vi "Configure Continuity.vi"(0 "VISA resource name":refnum<visa-resource-name>, 5 "Threshold (10)":dbl=10.0, 11 "error in (no error)":errorcluster) -> (4 "VISA resource name out":refnum<visa-resource-name>, 15 "error out":errorcluster)   [LabVIEW 2020, in "Keithley 27XX.lvlib"]
doc: "This VI configures the hreshold for continuity measurements.\n\nNote: \n(1) Configure Measurement.vi must be called <B>before</B> setting the threshold.\n\n(2) This VI will only work in Continuity Measurement mode.\n\n(3) This VI configures a global setting. Therefore, this VI does not require a scan list."
uses:
  Keithley 27XX.lvlib
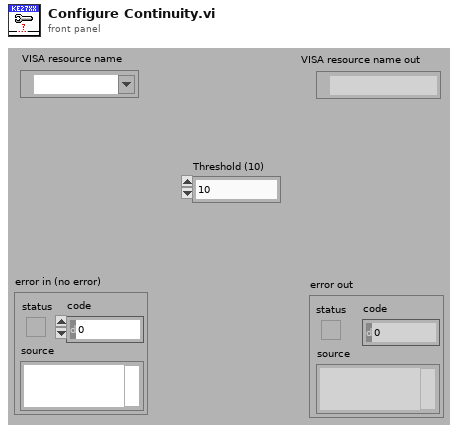
[diagram p1: front panel]
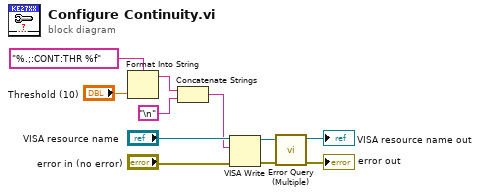
[diagram p0: block diagram]
diagram:
  n1 = Format Into String(format string="%.;:CONT:THR %f", "Threshold (10)") -> (resulting string=w2:string)  [unwired: 2 in, 1 out]
  n2 = Concatenate Strings(w2, "\n") -> (w1:string)
  n3 = VISA Write(VISA resource name="VISA resource name", write buffer=w1, error in (no error)="error in (no error)") -> (VISA resource name out=w7:refnum<visa-resource-name>, error out=w6:errorcluster)  [unwired: 1 out]
  n4 = call "Error Query (Multiple).vi"("VISA resource name"=w7, "error in (no error)"=w6) -> ("VISA resource name out"=→"VISA resource name out":refnum<visa-resource-name>, "error out"=→"error out":errorcluster)  [unwired: 10 in, 2 out]
